vi "KE622x -- 2182 -A Set NPLCs.vi"(0 "622x Resource In":refnum<visa-resource-name>, 1 "Check For SCPI Errors? (T)":bool=TRUE, 7 "2182 -A NPLCs":u32=5, 11 "error in (no error)":errorcluster) -> (4 "622x Resource Out (dupl)":refnum<visa-resource-name>, 15 "error out":errorcluster)   [LabVIEW 2013, in "Keithly user program.lvlib"]
uses:
  Keithly user program.lvlib
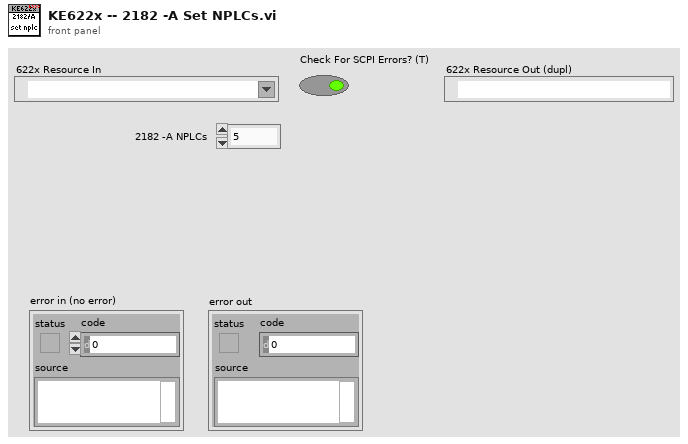
[diagram p1: front panel]
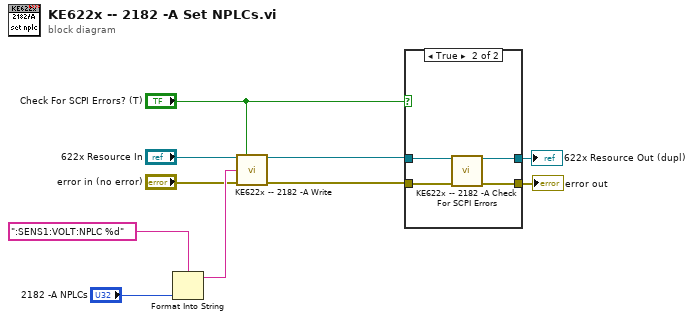
[diagram p0: block diagram]
diagram:
  n1 = Format Into String(format string=":SENS1:VOLT:NPLC %d", "2182 -A NPLCs") -> (resulting string=w3:string)  [unwired: 2 in, 1 out]
  n2 = call "KE622x -- 2182 -A Write.vi"("Resource In"="622x Resource In", "Check For SCPI Errors? (T)"="Check For SCPI Errors? (T)", "2182-A Write String"=w3, "error in (no error)"="error in (no error)") -> ("Resource Out (dupl)"=w5:refnum<visa-resource-name>, "error out"=w1:errorcluster)  [unwired: 10 in]
  n3 = case shown="True" "Check For SCPI Errors? (T)" {
    tunnel: w5 -> [w12 w16]
    tunnel: w1 -> [w11 w14]
    tunnel: [w12 w15] -> w10
    tunnel: [w11 w13] -> w9
    frame False {
    }
    frame True {
      n4 = call "KE622x -- 2182 -A Check For SCPI Errors.vi"("VISA Resource In"=w16, "error in (no error)"=w14) -> ("VISA Resource Out (dupl)"=w15:refnum<visa-resource-name>, "error out"=w13:errorcluster)  [unwired: 10 in, 2 out]
    }
  }
  "622x Resource Out (dupl)" <- w10
  "error out" <- w9
